vi "Control Labview.vi"() -> ()   [LabVIEW 2020]
uses:
  <vilib>/MakerHub/Xbox-One-Controller/Private/Type Defs/Indicators/Controller.ctl
  <vilib>/MakerHub/Xbox-One-Controller/Private/Type Defs/Indicators/A.ctl
  <vilib>/MakerHub/Xbox-One-Controller/Private/Type Defs/Indicators/B.ctl
  <vilib>/MakerHub/Xbox-One-Controller/Private/Type Defs/Indicators/X.ctl
  <vilib>/MakerHub/Xbox-One-Controller/Private/Type Defs/Indicators/Y.ctl
  <vilib>/MakerHub/Xbox-One-Controller/Private/Type Defs/Indicators/Left Bumper.ctl
  <vilib>/MakerHub/Xbox-One-Controller/Private/Type Defs/Indicators/Right Bumper.ctl
  <vilib>/MakerHub/Xbox-One-Controller/Private/Type Defs/Indicators/View.ctl
  <vilib>/MakerHub/Xbox-One-Controller/Private/Type Defs/Indicators/Menu.ctl
  <vilib>/MakerHub/Xbox-One-Controller/Private/Type Defs/Indicators/Thumbstick_Analog.ctl
  <vilib>/MakerHub/Xbox-One-Controller/Private/Type Defs/Indicators/Slider.ctl
  <vilib>/MakerHub/Xbox-One-Controller/Private/Type Defs/Indicators/DPad.ctl
  <vilib>/MakerHub/Xbox-One-Controller/Public/Open First Controller.vi
  <vilib>/MakerHub/Xbox-One-Controller/LMH-Xbox-One-Controller.lvlib
panel:
  out "millisecond timer value":u32
  out "Angle":dbl
  out "Y axis":dbl
  out "X axis":dbl
  out "Power":dbl
  out "Power":dbl(knob) scale=0.0..100.0
  in  "Stop Button":bool
  out "Controller":T1={"A Button"=FALSE, "B Button"=FALSE, "X Button"=FALSE, "Y Button"=FALSE, "Left Bumper"=FALSE, "Right Bumper"=FALSE, "View Button"=FALSE, "Menu Button"=FALSE, "Left Stick"={[], []}, "Right Stick"={[], []}, "Trigger"=0, "D-Pad"=5} {"Trigger" scale=32767.0..-32768.0}
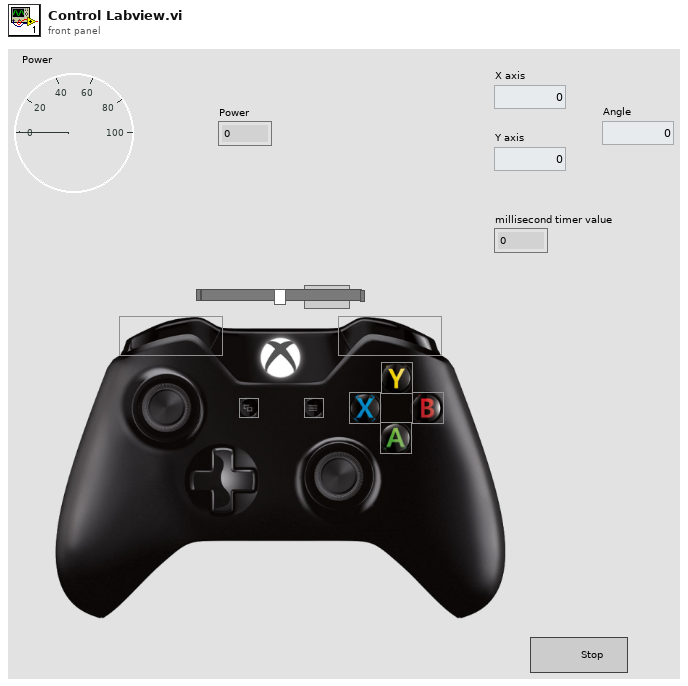
[diagram p1: front panel]
types:
  T1 = typedef "LMH-Xbox-One-Controller.lvlib/Controller.ctl" = cluster{"A Button":T2, "B Button":T3, "X Button":T4, "Y Button":T5, "Left Bumper":T6, "Right Bumper":T7, "View Button":T8, "Menu Button":T9, "Left Stick":T10, "Right Stick":T10, "Trigger":T11, "D-Pad":T12}
  T2 = typedef "LMH-Xbox-One-Controller.lvlib/A.ctl" = bool
  T3 = typedef "LMH-Xbox-One-Controller.lvlib/B.ctl" = bool
  T4 = typedef "LMH-Xbox-One-Controller.lvlib/X.ctl" = bool
  T5 = typedef "LMH-Xbox-One-Controller.lvlib/Y.ctl" = bool
  T6 = typedef "LMH-Xbox-One-Controller.lvlib/Left Bumper.ctl" = bool
  T7 = typedef "LMH-Xbox-One-Controller.lvlib/Right Bumper.ctl" = bool
  T8 = typedef "LMH-Xbox-One-Controller.lvlib/View.ctl" = bool
  T9 = typedef "LMH-Xbox-One-Controller.lvlib/Menu.ctl" = bool
  T10 = typedef "LMH-Xbox-One-Controller.lvlib/Thumbstick_Analog.ctl" = cluster{i32[], i32[]}
  T11 = typedef "LMH-Xbox-One-Controller.lvlib/Slider.ctl" = i32
  T12 = typedef "LMH-Xbox-One-Controller.lvlib/DPad.ctl" = u16
  T13 = typedef "LMH-Xbox-One-Controller.lvlib/Xbox One Controller Ref.ctl" = cluster{"Controller Ref":refnum<k1>, "Event Refnum":refnum<event-registration>, "Worker Ref":refnum<vi>}
  T14 = typedef "LMH-Xbox-One-Controller.lvlib/All Axis Data.ctl" = cluster{"Left Stick":cluster{"X Axis":i32, "Y Axis":i32}, "Right Stick":cluster{"X Axis":i32, "Y Axis":i32}, "Triggers":i32, "D-Pad":T15}
  T15 = typedef "LMH-Xbox-One-Controller.lvlib/DPad Enum.ctl" = enum16{"Idle", "Up", "Up / Right", "Right", "Down / Right", "Down", "Down / Left", "Left", "Up / Left"}
  T16 = typedef "LMH-Xbox-One-Controller.lvlib/All Buttons Visual.ctl" = cluster{"A":T2, "B":T3, "X":T4, "Y":T5, "Left Bumper":T6, "Right Bumper":T7, "View Button":T8, "Menu Button":T9, "Left Stick":T17, "Right Stick":T17}
  T17 = typedef "LMH-Xbox-One-Controller.lvlib/Thumbstick.ctl" = bool
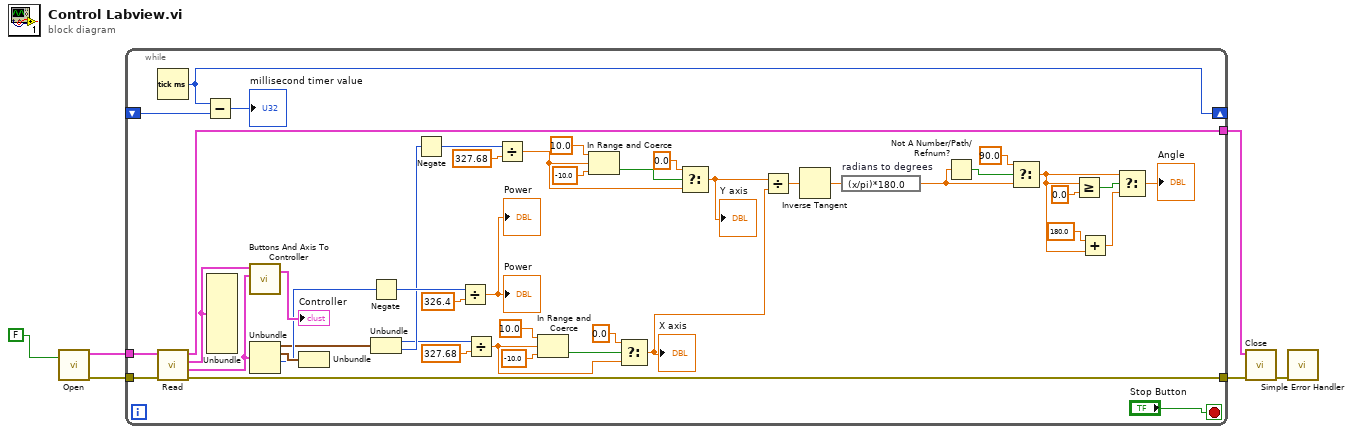
[diagram p0: block diagram]
diagram:
  n1 = call-poly <vilib>:"Open.vi"("Enable Events (T)"=FALSE) -> ("Error Out"=w3:errorcluster, "Xbox One Controller"=w2:T13)  [unwired: 8 in, 1 out]
  n2 = while {
    tunnel: w3 -> [w50]
    tunnel: w2 -> [w46]
    tunnel: [w49] -> w6
    tunnel: [w48] -> w5
    shift-right: [w9] -> _
    shift-left: _ -> [w8]
    stop <- "Stop Button" stop-if-true
    n3 = Tick Count (ms)() -> (millisecond timer value=w9:u32)
    n4 = call <vilib>:"Read.vi"("Error In"=w50, "Xbox One Controller Ref"=w46) -> ("Error Out"=w48:errorcluster, "All Axis"=w44:T14, "Buttons"=w45:T16, "Xbox One Controller Ref"=w49:T13)  [unwired: 6 in]
    n5 = Subtract(x=w9, y=w8) -> (x-y=→"millisecond timer value":u32)
    n6 = Unbundle(w45) -> ()  [unwired: 10 out]
    n7 = call <vilib>:"Buttons And Axis To Controller.vi"("All Axis"=w44, "Buttons"=w45) -> ("Controller"=→"Controller":T1)  [unwired: 5 in]
    n8 = Unbundle(w44) -> ("Left Stick"=w38:cluster{"X Axis":i32, "Y Axis":i32}, "Right Stick"=w43:cluster{"X Axis":i32, "Y Axis":i32}, "Triggers"=w42:i32)  [unwired: 1 out]
    n9 = Unbundle(w43) -> ()  [unwired: 2 out]
    n10 = Negate(x=w42) -> (-x=w41:i32)
    n11 = Unbundle(w38) -> ("X Axis"=w20:i32, "Y Axis"=w34:i32)
    n12 = Negate(x=w34) -> (-x=w36:i32)
    n13 = Divide(x=w41, y=326.4) -> (x/y=→"Power" →"Power":dbl)
    n14 = Divide(x=w20, y=327.68) -> (x/y=w29:dbl)
    n15 = Divide(x=w36, y=327.68) -> (x/y=w24:dbl)
    n16 = In Range and Coerce(upper limit=10.0, x=w29, lower limit=-10.0) -> (In Range?=w31:bool)  [unwired: 1 out]
    n17 = In Range and Coerce(upper limit=10.0, x=w24, lower limit=-10.0) -> (In Range?=w26:bool)  [unwired: 1 out]
    n18 = Select(t=0.0, s=w31, f=w29) -> (s? t:f=w22:dbl)
    "X axis" <- w22
    n19 = Select(t=0.0, s=w26, f=w24) -> (s? t:f=w23:dbl)
    "Y axis" <- w23
    n20 = Divide(x=w23, y=w22) -> (x/y=w17:dbl)
    n21 = Inverse Tangent(1:w17) -> (0:w21:dbl)
    n22 = expression code="(x/pi)*180.0" "radians to degrees"(w21) -> (w16:dbl)
    n23 = Not A Number/Path/Refnum?(number/path/refnum=w16) -> (NaN/Path/Refnum?=w19:bool)
    n24 = Select(t=90.0, s=w19, f=w16) -> (s? t:f=w11:dbl)
    n25 = Greater Or Equal?(x=w11, y=0.0) -> (x >= y?=w14:bool)
    n26 = Add(x=180.0, y=w11) -> (x+y=w13:dbl)
    n27 = Select(t=w11, s=w14, f=w13) -> (s? t:f=→"Angle":dbl)
  }
  n28 = call <vilib>:"Close.vi"("Error In"=w5, "Xbox One Controller Ref"=w6) -> ("Error Out"=w4:errorcluster)  [unwired: 9 in]
  n29 = call <vilib>:"Simple Error Handler.vi"("error in (no error)"=w4) -> ()  [unwired: 4 in, 5 out]
